vi "Reverse Data Set V2.vi"(9 "Pos to Start Scan":i32=10000, 10 "data value reference":refnum<data-value>, 11 "Final No of Blocks":i32) -> (2 "data value ref out":refnum<data-value>)   [LabVIEW 2015, in "Tool Module.lvlib"]
uses:
  Tool Module.lvlib
  ToolModGLOB.vi
  Tool Config/Tool Cfg.lvlib
panel:
  out "Sample Count Graph":u32[](graph)
  out "Axial Pos Array":dbl[](array[numeric])
  out "Reversed Array out":u32[][](array[numeric])
  in  "Scan Data Array in":u32[][](array[numeric])=[[0, 1, 2, 3, 4, 5], [10, 11, 12, 13, 14, 15], [20, 21, 22, 23, 24, 25], [30, 31, 32, 33, 34, 35], [40, 41, 42, 43, 44, 45]]
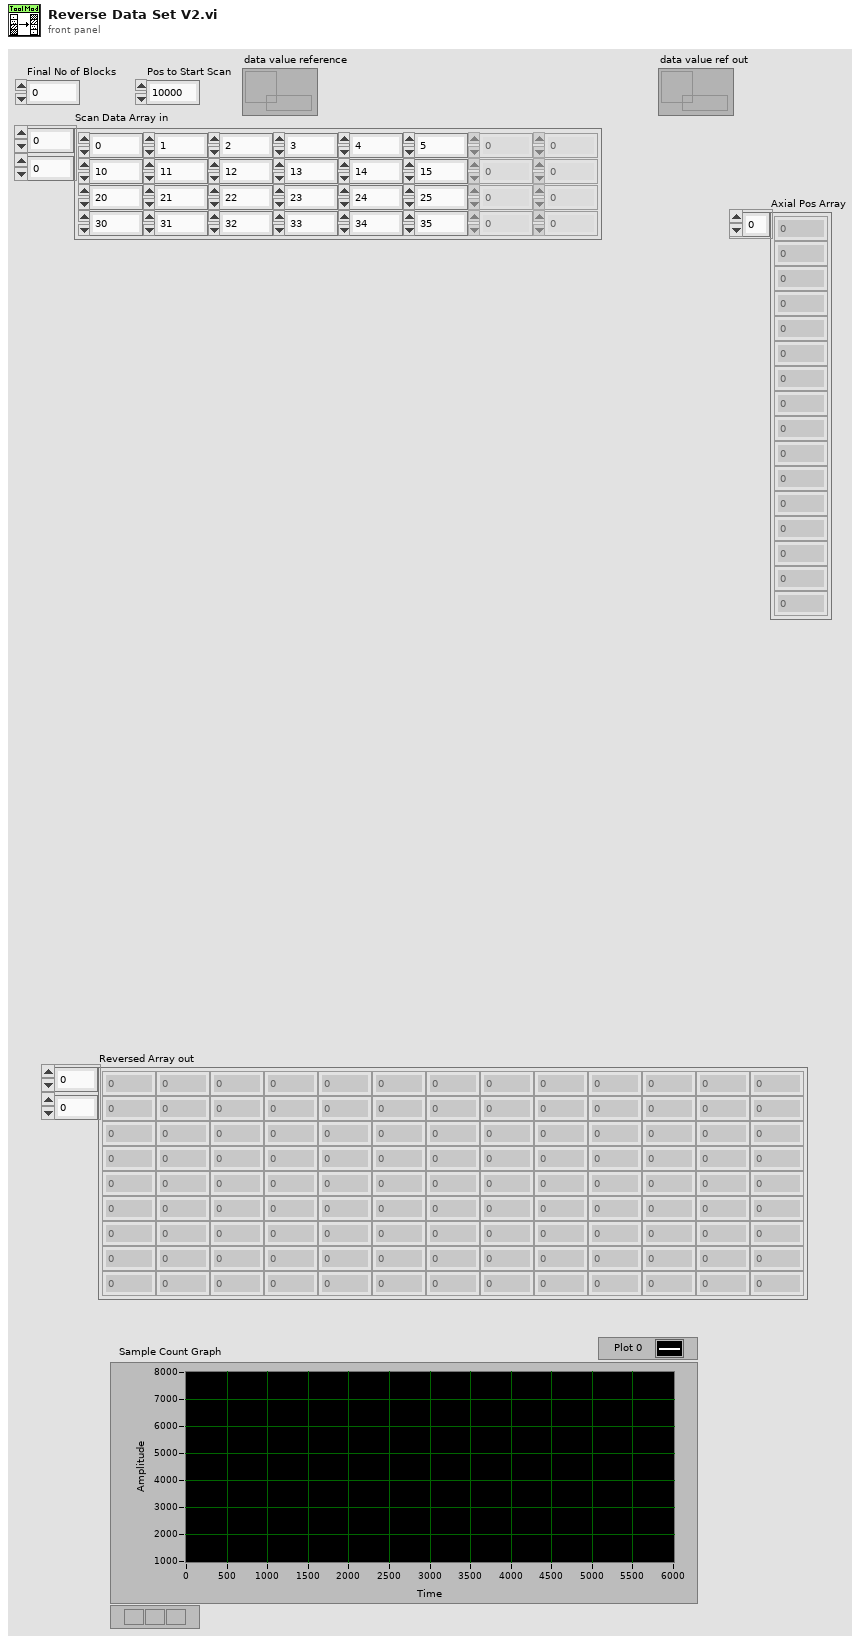
[diagram p1: front panel]
types:
  T1 = typedef "_Data Stream Fmt Params Cluster--typedef.ctl" = cluster{"Samples per Block":i32, "Raw Data Status Len":i32, "Fltr Data Status Len":i32}
  T2 = typedef "Tool Cfg.lvlib/_Tool Operation Config Cluster--typedef.ctl" = cluster{"Use Tool Cfg":bool, "Use Tool Cal":bool, "Fake Data?":bool, "Mode":i16, "Array Subset Length":i16, "nArrays to Read":i16, "Full Array Read Length":i16, "nSubarrays/Sensor":i16}
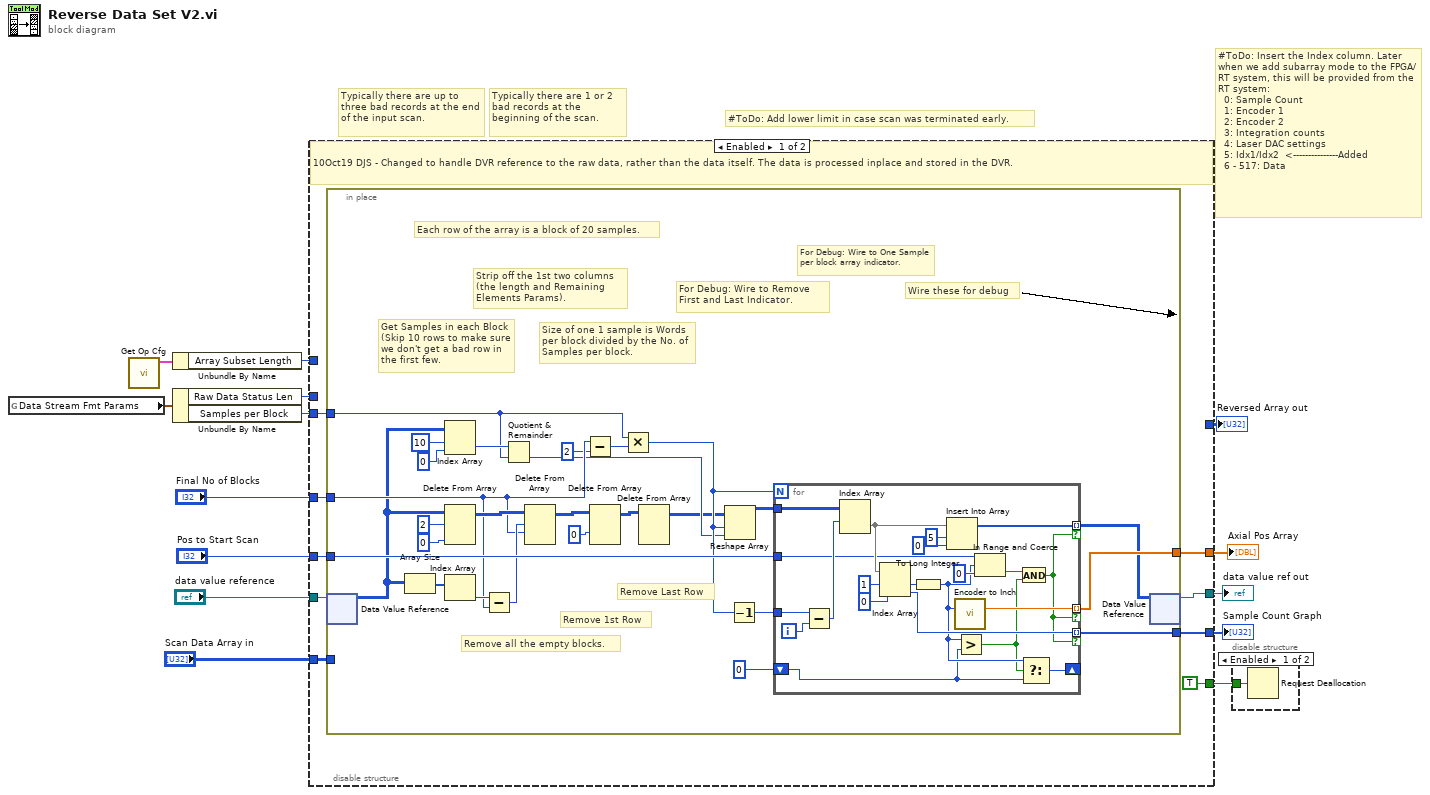
[diagram p0: block diagram]
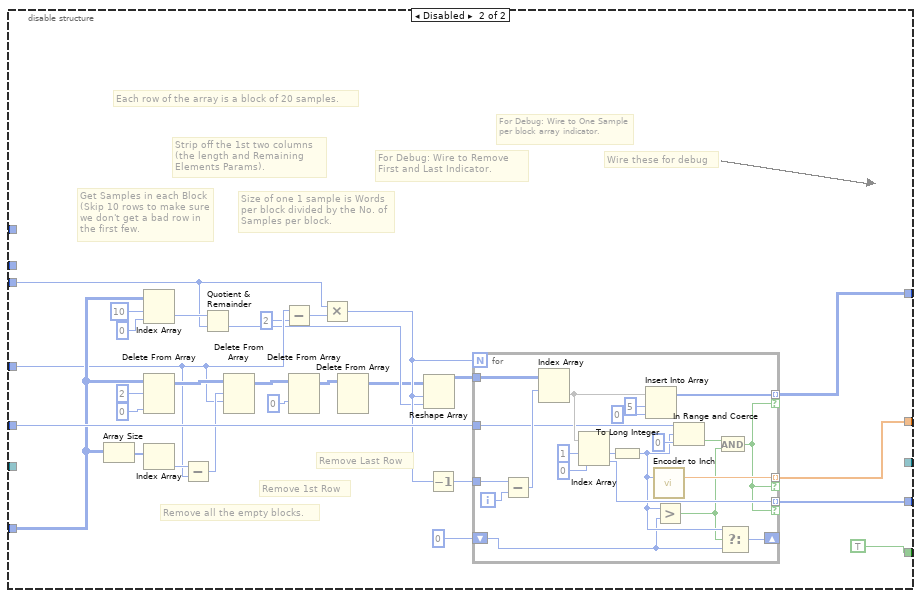
[diagram p2: hidden frame]
diagram:
  # "#ToDo: Insert the Index column. Later when we add subarray mode to the FPGA/RT system, this will be provided from the RT system:\n  0: Sample Count\n  1: Encoder 1\n  2: Encoder 2\n  3: Integration counts\n  4: Laser DAC settings\n  5: Idx1/Idx2  <---------------Added\n  6 - 517: Data"
  # "#ToDo: Add lower limit in case scan was terminated early."
  # "Typically there are 1 or 2 bad records at the beginning of the scan."
  # "Typically there are up to three bad records at the end of the input scan."
  n1 = global read "ToolModGLOB.vi" "Data Stream Fmt Params"() -> (w13:T1)
  n2 = call "Get Op Cfg.vi"() -> ("Tool Operation Config"=w11:T2)  [unwired: 11 in]
  n3 = Unbundle By Name(w11) -> ("Array Subset Length"=w10:i16)
  n4 = Unbundle By Name(w13) -> ("Raw Data Status Len"=w12:i32, "Samples per Block"=w9:i32)
  n5 = disable-structure shown="Enabled" {
    disable-tunnel: "Final No of Blocks" -> [w21 w85]
    disable-tunnel: "Scan Data Array in" -> [w22 w91]
    disable-tunnel: w12 -> [_ _]
    disable-tunnel: w10 -> [_ _]
    disable-tunnel: w9 -> [w20 w83]
    disable-tunnel: "Pos to Start Scan" -> [w23 w93]
    disable-tunnel: [_ w81] -> w7
    disable-tunnel: [w18 w73] -> w5
    disable-tunnel: [w19 w74] -> w4
    disable-tunnel: [TRUE TRUE] -> w3
    disable-tunnel: "data value reference" -> [w15 _]
    disable-tunnel: [w16 _] -> w1
    frame Enabled {
      # "10Oct19 DJS - Changed to handle DVR reference to the raw data, rather than the data itself. The data is processed inplace and stored in the DVR."
      n6 = in-place {
        in-place-border: w23 -> [w44]
        in-place-border: w22 -> [_]
        in-place-border: w21 -> [w37]
        in-place-border: w20 -> [w35]
        in-place-border: [w27] -> w19
        in-place-border: [w26] -> w18
        # "Each row of the array is a block of 20 samples."
        # "Size of one 1 sample is Words per block divided by the No. of Samples per block."
        # "Get Samples in each Block (Skip 10 rows to make sure we don't get a bad row in the first few."
        # "Remove all the empty blocks."
        # "Strip off the 1st two columns (the length and Remaining Elements Params)."
        # "For Debug: Wire to One Sample per block array indicator."
        # "For Debug: Wire to Remove First and Last Indicator."
        # "Wire these for debug"
        # "Remove Last Row"
        # "Remove 1st Row"
        n7 = in-place-dvr #1(w15) -> (w25:u32[][])  [unwired: 1 out]
        n8 = Array Size(array=w25) -> (size(s)=w42:i32[])
        n9 = Index Array(array=w25, index (row)=10, index (col)=0 ("disabled index (col)")) -> (element=w50:u32)
        n10 = Delete From Array(array=w25, length=2, index (col)=0 ("disabled index (col)")) -> (array with subset deleted=w43:u32[][])  [unwired: 1 in, 1 out]
        n11 = Index Array(array=w42) -> (element=w41:i32)  [unwired: 1 in]
        n12 = Subtract(x=w41, y=w37) -> (x-y=w40:i32)
        n13 = Quotient & Remainder(x=w50, y=w35) -> (floor(x/y)=w30:u32)  [unwired: 1 out]
        n14 = Delete From Array(array=w43, length=w40, index (row)=w37) -> (array with subset deleted=w34:u32[][])  [unwired: 1 in, 1 out]
        n15 = Subtract(x=w37, y=2) -> (x-y=w32:i32)
        n16 = Delete From Array(array=w34, index (row)=0) -> (array with subset deleted=w38:u32[][])  [unwired: 2 in, 1 out]
        n17 = Multiply(x=w35, y=w32) -> (x*y=w31:i32)
        n18 = Delete From Array(array=w38) -> (array with subset deleted=w28:u32[][])  [unwired: 3 in, 1 out]
        n19 = Reshape Array(w28, w31, w30) -> (w33:u32[][])
        n20 = Decrement(x=w31) -> (x-1=w45:i32)
        n21 = for {
          N: w31 -> [_]
          tunnel: w33 -> [w71]
          tunnel: w45 -> [w68]
          tunnel: [w61] -> w24 mode=indexing if=w52
          tunnel: w44 -> [w63]
          tunnel: [w64] -> w27 mode=indexing if=w52
          tunnel: [w57] -> w26 mode=indexing if=w52
          shift-right: [w55] -> _
          shift-left: 0 -> [w53]
          i -> [w69]
          n22 = Subtract(x=w68, y=w69) -> (x-y=w70:i32)
          n23 = Index Array(array=w71, index (row)=w70) -> (element=w67:u32[])  [unwired: 1 in]
          n24 = Index Array(array=w67, index #1=1 ("index"), index #2=0 ("index")) -> (element #1=w66:u32, element #2=w57:u32)
          n25 = To Long Integer(number=w66) -> (32bit integer=w54:i32)
          n26 = Insert Into Array(array=w67, index=5, new element=u32 0 ("new element/subarray")) -> (w61:u32[])
          n27 = call "Encoder to Inch.vi"("Encoder in"=w54) -> ("Encoder out(in)"=w64:dbl)  [unwired: 14 in]
          n28 = Greater?(x=w54, y=w53) -> (0:w51:bool)
          n29 = In Range and Coerce(upper limit=w63, x=w54, lower limit=0) -> (In Range?=w56:bool)  [unwired: 1 out]
          n30 = And(x=w56, y=w51) -> (x .and. y?=w52:bool)
          n31 = Select(t=w54, s=w51, f=w53) -> (s? t:f=w55:i32)
        }
        n32 = in-place-dvr #1(w24) -> (w16:refnum<data-value>)  [unwired: 1 out]
      }
    }
    frame Disabled {
      # "Each row of the array is a block of 20 samples."
      # "Size of one 1 sample is Words per block divided by the No. of Samples per block."
      # "Get Samples in each Block (Skip 10 rows to make sure we don't get a bad row in the first few."
      # "Remove all the empty blocks."
      # "Strip off the 1st two columns (the length and Remaining Elements Params)."
      # "For Debug: Wire to One Sample per block array indicator."
      # "For Debug: Wire to Remove First and Last Indicator."
      # "Wire these for debug"
      # "Remove Last Row"
      # "Remove 1st Row"
      n33 = Array Size(array=w91) -> (size(s)=w90:i32[])
      n34 = Index Array(array=w91, index (row)=10, index (col)=0 ("disabled index (col)")) -> (element=w99:u32)
      n35 = Delete From Array(array=w91, length=2, index (col)=0 ("disabled index (col)")) -> (array with subset deleted=w92:u32[][])  [unwired: 1 in, 1 out]
      n36 = Index Array(array=w90) -> (element=w89:i32)  [unwired: 1 in]
      n37 = Subtract(x=w89, y=w85) -> (x-y=w88:i32)
      n38 = Quotient & Remainder(x=w99, y=w83) -> (floor(x/y)=w77:u32)  [unwired: 1 out]
      n39 = Delete From Array(array=w92, length=w88, index (row)=w85) -> (array with subset deleted=w82:u32[][])  [unwired: 1 in, 1 out]
      n40 = Subtract(x=w85, y=2) -> (x-y=w79:i32)
      n41 = Delete From Array(array=w82, index (row)=0) -> (array with subset deleted=w86:u32[][])  [unwired: 2 in, 1 out]
      n42 = Multiply(x=w83, y=w79) -> (x*y=w78:i32)
      n43 = Delete From Array(array=w86) -> (array with subset deleted=w75:u32[][])  [unwired: 3 in, 1 out]
      n44 = Reshape Array(w75, w78, w77) -> (w80:u32[][])
      n45 = Decrement(x=w78) -> (x-1=w94:i32)
      n46 = for {
        N: w78 -> [_]
        tunnel: w80 -> [w120]
        tunnel: w94 -> [w117]
        tunnel: [w110] -> w81 mode=indexing if=w101
        tunnel: w93 -> [w112]
        tunnel: [w113] -> w74 mode=indexing if=w101
        tunnel: [w106] -> w73 mode=indexing if=w101
        shift-right: [w104] -> _
        shift-left: 0 -> [w102]
        i -> [w118]
        n47 = Subtract(x=w117, y=w118) -> (x-y=w119:i32)
        n48 = Index Array(array=w120, index (row)=w119) -> (element=w116:u32[])  [unwired: 1 in]
        n49 = Index Array(array=w116, index #1=1 ("index"), index #2=0 ("index")) -> (element #1=w115:u32, element #2=w106:u32)
        n50 = To Long Integer(number=w115) -> (32bit integer=w103:i32)
        n51 = Insert Into Array(array=w116, index=5, new element=u32 0 ("new element/subarray")) -> (w110:u32[])
        n52 = call "Encoder to Inch.vi"("Encoder in"=w103) -> ("Encoder out(in)"=w113:dbl)  [unwired: 14 in]
        n53 = Greater?(x=w103, y=w102) -> (0:w100:bool)
        n54 = In Range and Coerce(upper limit=w112, x=w103, lower limit=0) -> (In Range?=w105:bool)  [unwired: 1 out]
        n55 = And(x=w105, y=w100) -> (x .and. y?=w101:bool)
        n56 = Select(t=w103, s=w100, f=w102) -> (s? t:f=w104:i32)
      }
    }
  }
  "Reversed Array out" <- w7
  "Axial Pos Array" <- w4
  "Sample Count Graph" <- w5
  "data value ref out" <- w1
  n57 = disable-structure shown="Enabled" {
    disable-tunnel: w3 -> [w121 _]
    frame Enabled {
      n58 = Request Deallocation(w121) -> ()
    }
    frame Disabled {
    }
  }
